vi "p1.vi"() -> ()   [LabVIEW 2021, in "d9.lvlib"]
uses:
  d9.lvlib
  <userlib>/_OpenG.lib/array/array.llb/Remove Duplicates from 1D Array (Variant)__ogtk.vi
  AOC/AOC.lvlib
panel:
  in  "Example":string="R 4\nU 4\nL 3\nD 1\nR 4\nD 1\nL 5\nR 2"
  in  "Example":bool
  out "Answer":i64=6498
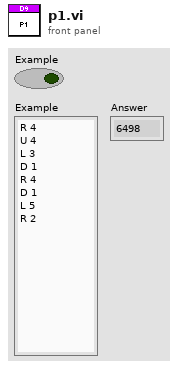
[diagram p1: front panel]
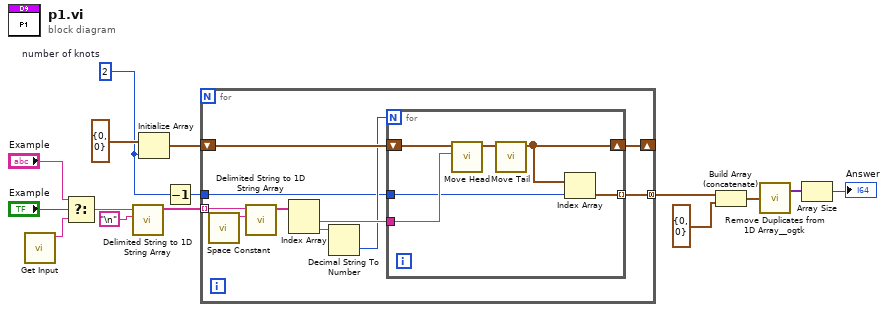
[diagram p0: block diagram]
diagram:
  w2 = 2  # number of knots
  n1 = call "Get Input.vi"() -> ("Input"=w15:string)  [unwired: 11 in]
  n2 = Select(t="Example", s="Example", f=w15) -> (s? t:f=w14:string)
  n3 = call <vilib>:"Delimited String to 1D String Array.vi"("delimiter"="\n", "delimited string"=w14) -> ("string array"=w10:string[])  [unwired: 9 in]
  n4 = Initialize Array(cluster{"x":i64, "y":i64} {"x"=0, "y"=0} ("Knot"), w2) -> (w3:cluster{"x":i64, "y":i64}[])
  n5 = Decrement(x=w2) -> (x-1=w1:i32)
  n6 = for {
    tunnel: w10 -> [w25] mode=indexing
    shift-right: [w20] -> _
    shift-left: w3 -> [w21]
    tunnel: [w19] -> w9 mode=concatenating
    tunnel: w1 -> [w16]
    n7 = call <vilib>:"Space Constant.vi"() -> ("String"=w24:string)
    n8 = call <vilib>:"Delimited String to 1D String Array.vi"("delimiter"=w24, "delimited string"=w25) -> ("string array"=w23:string[])  [unwired: 9 in]
    n9 = Index Array(array=w23) -> (element #1=w22:string, element #2=w18:string)  [unwired: 2 in]
    n10 = Decimal String To Number(string=w18) -> (number=w17:i32)  [unwired: 2 in, 1 out]
    n11 = for {
      N: w17 -> [_]
      tunnel: w22 -> [w29]
      tunnel: [w27] -> w19 mode=indexing
      shift-right: [w28] -> w20
      shift-left: w21 -> [w30]
      tunnel: w16 -> [w26]
      n12 = call "Move Head.vi"("Direction"=w29, "Rope in"=w30) -> ("Rope out"=w31:cluster{"x":i64, "y":i64}[])  [unwired: 9 in]
      n13 = call "Move Tail.vi"("Rope in"=w31) -> ("Rope out"=w28:cluster{"x":i64, "y":i64}[])  [unwired: 10 in]
      n14 = Index Array(array=w28, index=w26) -> (element=w27:cluster{"x":i64, "y":i64})
    }
  }
  n15 = Build Array (concatenate)(w9, cluster{"x":i64, "y":i64} {"x"=0, "y"=0} ("element")) -> (w7:cluster{"x":i64, "y":i64}[])
  n16 = call-poly <userlib>:"Remove Duplicates from 1D Array__ogtk.vi"("Input Array"=w7) -> ("Output Array"=w6:variant[])  [unwired: 1 out]
  n17 = Array Size(array=w6) -> (size(s)=→"Answer":i32)
